vi "Array_2D parametric sorting.vi"(9 "Order (ascending)":enum16{"Ascending", "Descending"}(ring), 10 "Priority Columns (1,0)":i32[](array[numeric]), 11 "Unsorted Array":dbl[][](array[numeric])) -> (1 "Sorted Pointers":i32[](array[numeric]), 3 "Sorted Array":dbl[][](array[numeric]))   [LabVIEW 2020]
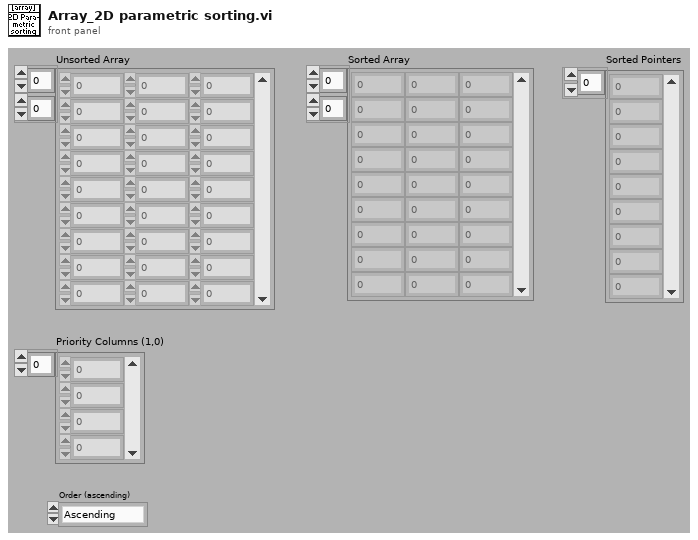
[diagram p1: front panel]
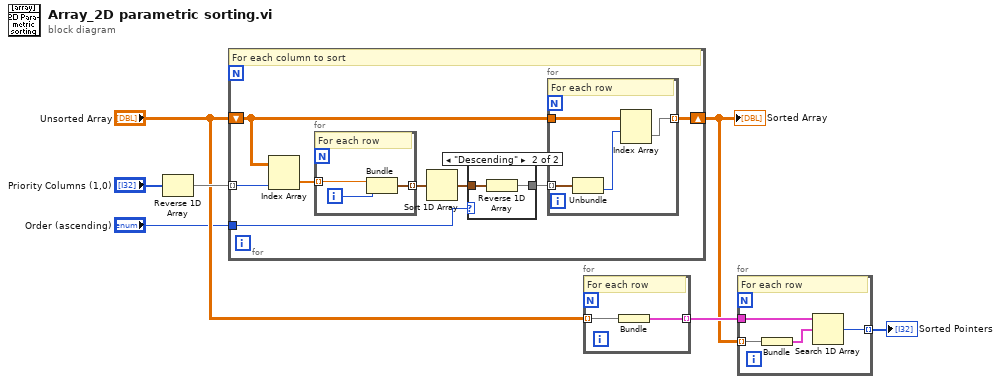
[diagram p0: block diagram]
diagram:
  n1 = Reverse 1D Array(array="Priority Columns (1,0)") -> (reversed array=w7:i32[])
  n2 = for {
    shift-right: [w9] -> w3
    shift-left: "Unsorted Array" -> [w11]
    tunnel: w7 -> [w8] mode=indexing
    tunnel: "Order (ascending)" -> [w10]
    # "For each column to sort"
    n3 = Index Array(array=w11, index (col)=w8) -> (element=w13:dbl[])  [unwired: 1 in]
    n4 = for {
      tunnel: w13 -> [w23] mode=indexing
      tunnel: [w25] -> w12 mode=indexing
      i -> [w24]
      # "For each row"
      n5 = Bundle("number: 0 to 1"=w23, w24) -> (w25:cluster{"number: 0 to 1":dbl, i32})  [unwired: 1 out]
    }
    n6 = Sort 1D Array(array=w12) -> (sorted array=w15:cluster{"number: 0 to 1":dbl, i32}[])
    n7 = case shown="\"Descending\"" w10 {
      tunnel: [w16 w17] -> w14
      tunnel: w15 -> [w16 w18]
      frame "Ascending", Default {
      }
      frame "Descending" {
        n8 = Reverse 1D Array(array=w18) -> (reversed array=w17:cluster{"number: 0 to 1":dbl, i32}[])
      }
    }
    n9 = for {
      tunnel: w14 -> [w22] mode=indexing
      tunnel: w11 -> [w21]
      tunnel: [w19] -> w9 mode=indexing
      # "For each row"
      n10 = Unbundle(w22) -> (w20:i32)  [unwired: 1 out]
      n11 = Index Array(array=w21, index (row)=w20) -> (element=w19:dbl[])  [unwired: 1 in]
    }
  }
  "Sorted Array" <- w3
  n12 = for {
    tunnel: "Unsorted Array" -> [w27] mode=indexing
    tunnel: [w26] -> w6 mode=indexing
    # "For each row"
    n13 = Bundle("Unsorted Array"=w27) -> (w26:cluster{"Unsorted Array":dbl[]})  [unwired: 1 in]
  }
  n14 = for {
    tunnel: w3 -> [w30] mode=indexing
    tunnel: w6 -> [w31]
    tunnel: [w28] -> w5 mode=indexing
    # "For each row"
    n15 = Bundle("Unsorted Array"=w30) -> (w29:cluster{"Unsorted Array":dbl[]})  [unwired: 1 in]
    n16 = Search 1D Array(1D array=w31, element=w29) -> (index of element=w28:i32)  [unwired: 1 in]
  }
  "Sorted Pointers" <- w5
